vi "Init.vi"(10 "Output":refnum<data-value>) -> (3 "TEMPLATE Msg Output":refnum<class "TEMPLATE Msg Output.lvclass">)   [LabVIEW 2020, in "_Template.lvlib" / "Templates.lvlib" / "TEMPLATE jettl Msg.lvlib" / "TEMPLATE Msg Output.lvclass"]
uses:
  TEMPLATE Msg Output.lvclass
  TEMPLATE Msg Output.lvclass/TEMPLATE Msg Output.ctl
  Output.ctl
  TEMPLATE jettl Msg.lvlib
panel:
  # "This front panel should not be manipulated."
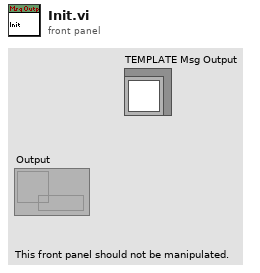
[diagram p1: front panel]
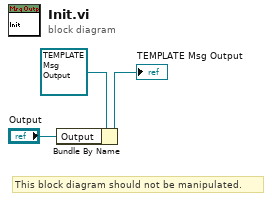
[diagram p0: block diagram]
diagram:
  # "This block diagram should not be manipulated."
  n1 = Bundle By Name(cluster=refnum<class "TEMPLATE Msg Output.lvclass"> refnum ("TEMPLATE Msg Output"), "Output"="Output") -> (→"TEMPLATE Msg Output":refnum<class "TEMPLATE Msg Output.lvclass">)
